vi "Close.vi"(8 "error in":errorcluster, 11 "Fgen Base in":refnum<class "Fgen Base.lvclass">) -> (0 "error out":errorcluster, 3 "Fgen Base out":refnum<class "Fgen Base.lvclass">)   [LabVIEW 2023, in "Fgen Base.lvlib" / "Fgen Base.lvclass"]
uses:
  Fgen Base.lvclass
  Fgen Base.lvclass/Fgen Base.ctl
  Interfaces/IConfigure/IConfigure.lvclass
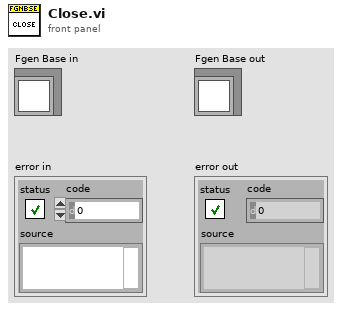
[diagram p1: front panel]
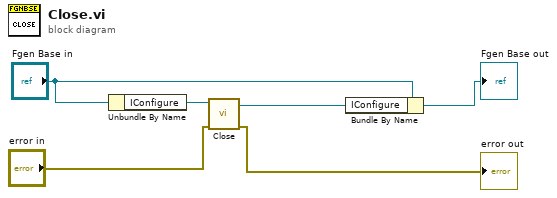
[diagram p0: block diagram]
diagram:
  n1 = Unbundle By Name("Fgen Base in") -> ("IConfigure"=w6:refnum<class "IConfigure.lvclass">)
  n2 = call-dynamic "Close.vi"("error in"="error in", "IConfigure in"=w6) -> ("error out"=→"error out":errorcluster, "IConfigure out"=w1:refnum<class "IConfigure.lvclass">)  [unwired: 8 in]
  n3 = Bundle By Name(cluster="Fgen Base in", "IConfigure"=w1) -> (→"Fgen Base out":refnum<class "Fgen Base.lvclass">)
